vi "Compressor Config.vi"(9 "Relay Channel":T1, 11 "Pressure Switch DIO Channel":T2) -> ()   [LabVIEW 2012]
uses:
  <vilib>/Rock Robotics/SystemInterfaces/DIO/FPGA_DIOChannel.ctl
  <vilib>/Rock Robotics/SystemInterfaces/DIO/FPGA_DIORelayChannel.ctl
  <vilib>/Rock Robotics/WPI/Compressor/WPI_CompressorGetSetRefNum.vi
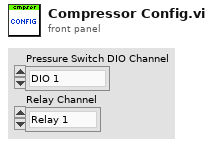
[diagram p1: front panel]
types:
  T1 = typedef "FPGA_DIORelayChannel.ctl" = enum8{"Relay 1", "Relay 2", "Relay 3", "Relay 4", "Relay 5", "Relay 6", "Relay 7", "Relay 8", "Invalid"}
  T2 = typedef "FPGA_DIOChannel.ctl" = enum8{"DIO 1", "DIO 2", "DIO 3", "DIO 4", "DIO 5", "DIO 6", "DIO 7", "DIO 8", "DIO 9", "DIO 10", "DIO 11", "DIO 12", "DIO 13", "DIO 14", "Invalid"}
  T3 = typedef "WPI_CompressorDevRef.ctl" = cluster{"DevStatus":errorcluster, "DigitalInputDevRef":T4, "RelayDevRef":T6}
  T4 = typedef "WPI_DigitalInputDevRef.ctl" = cluster{"DevStatus":errorcluster, "DIO Channel":T2, "Digital Module":T5}
  T5 = typedef "FPGA_TypedefDigitalModule.ctl" = enum16{"Digital Module 1", "Digital Module 2"}
  T6 = typedef "WPI_RelayDevRef.ctl" = cluster{"DevStatus":errorcluster, "Relay Channel":T1, "Digital Module":T5, "Relay Direction":T7}
  T7 = typedef "WPI_RelayDirection.ctl" = enum16{"Both directions", "Forward only", "Reverse only"}
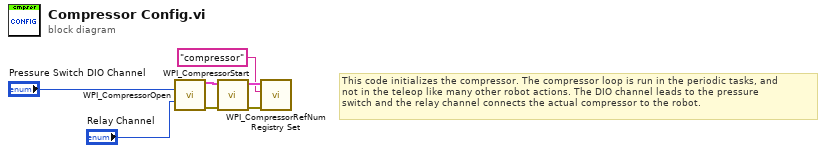
[diagram p0: block diagram]
diagram:
  # "This code initializes the compressor. The compressor loop is run in the periodic tasks, and \nnot in the teleop like many other robot actions. The DIO channel leads to the pressure\nswitch and the relay channel connects the actual compressor to the robot."
  n1 = call <vilib>:"WPI_CompressorOpen.vi"("Pressure Switch DIO Channel"="Pressure Switch DIO Channel", "Relay Channel"="Relay Channel") -> ("CompressorDevRef"=w7:T3, "error out"=w6:errorcluster)  [unwired: 12 in]
  n2 = call <vilib>:"WPI_CompressorStart.vi"("error in (no error)"=w6, "CompressorDevRef"=w7) -> ("error out"=w4:errorcluster, "CompressorDevRef"=w5:T3)  [unwired: 8 in]
  n3 = call <vilib>:"WPI_CompressorRefNum Registry Set.vi"("error in (no error)"=w4, "refnum name"="compressor", "CompressorDevRef"=w5) -> ()  [unwired: 7 in, 2 out]
